vi "finding_high_and_low.vi"() -> ()   [LabVIEW 2019]
uses:
  Control.ctl
panel:
  in  "Stop":bool
  in  "Interrupt":bool
  out "Too low":bool
  out "Good":bool
  out "Too high":bool
  out "Value":dbl
  in  "Start":bool
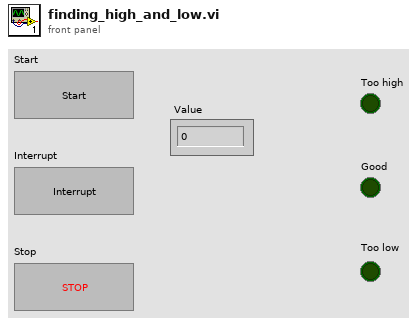
[diagram p1: front panel]
types:
  T1 = typedef "Control.ctl" = enum16{"measurment", "Good", "Too Low", "Too High", "End", "wait", "Pause"}
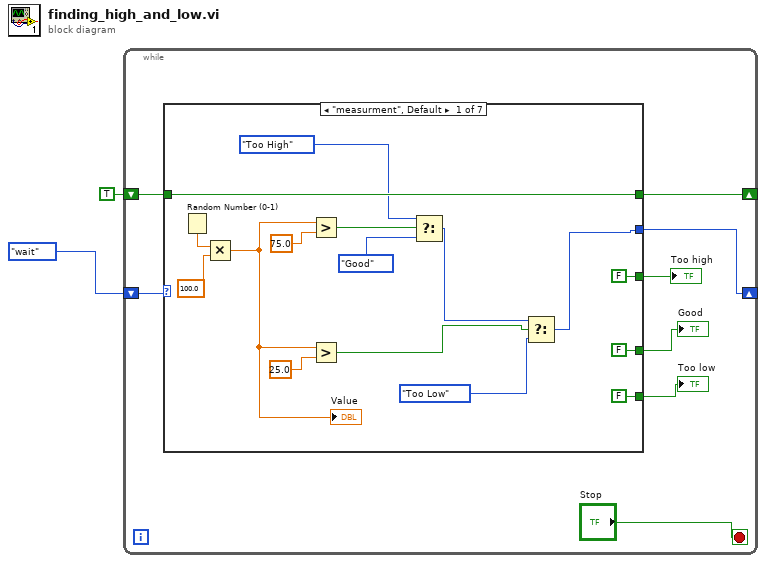
[diagram p0: block diagram]
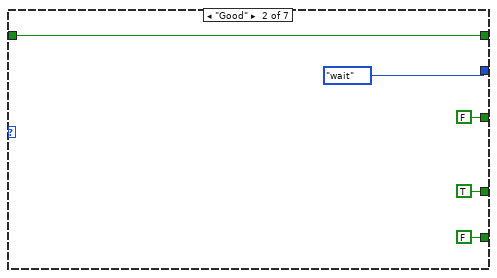
[diagram p2: hidden frame]
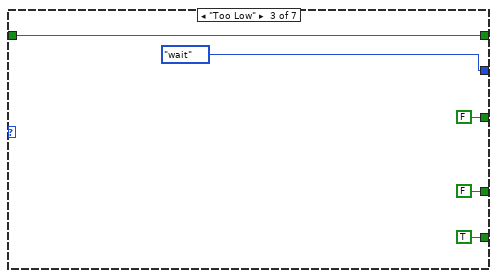
[diagram p3: hidden frame]
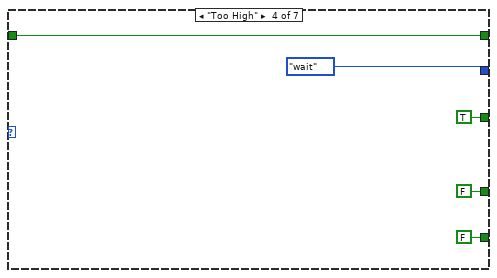
[diagram p4: hidden frame]
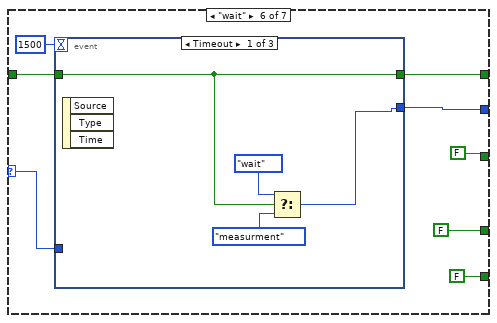
[diagram p6: hidden frame]
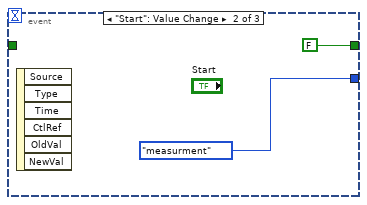
[diagram p7: hidden frame]
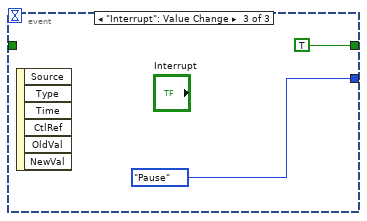
[diagram p8: hidden frame]
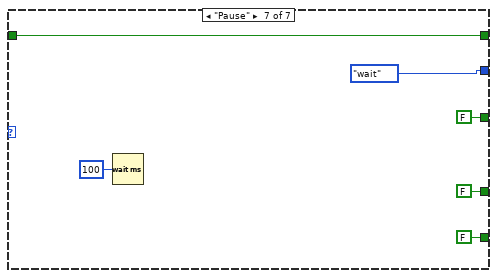
[diagram p9: hidden frame]
diagram:
  n1 = while {
    shift-right: [w9] -> _
    shift-left: Control."wait" -> [w10]
    shift-right: [w7] -> _
    shift-left: TRUE -> [w6]
    stop <- "Stop" stop-if-true
    n2 = case shown="\"measurment\", Default" w10 {
      selector: w10 -> [_ _ _ _ _ w44 _]
      tunnel: [w20 Control."wait" Control."wait" Control."wait" _ w50 Control."wait"] -> w9
      tunnel: [FALSE FALSE FALSE TRUE _ FALSE FALSE] -> w8
      tunnel: [w16 w31 w36 w41 w42 w48 w64] -> w7
      tunnel: w6 -> [w16 w31 w36 w41 w42 w47 w64]
      tunnel: [FALSE TRUE FALSE FALSE _ FALSE FALSE] -> w5
      tunnel: [FALSE FALSE TRUE FALSE _ FALSE FALSE] -> w4
      frame "measurment", Default {
        n3 = Random Number (0-1)() -> (number: 0 to 1=w12:dbl)
        n4 = Multiply(x=w12, y=100.0) -> (x*y=w13:dbl)
        "Value" <- w13
        n5 = Greater?(x=w13, y=75.0) -> (0:w23:bool)
        n6 = Greater?(x=w13, y=25.0) -> (0:w22:bool)
        n7 = Select(t=Control."Too High", s=w23, f=Control."Good") -> (s? t:f=w21:T1)
        n8 = Select(t=w21, s=w22, f=Control."Too Low") -> (s? t:f=w20:T1)
      }
      frame "Good" {
      }
      frame "Too Low" {
      }
      frame "Too High" {
      }
      frame "End" {
      }
      frame "wait" {
        n9 = event shown="[0] Timeout" {
          selector: _ -> [_ _ _]
          dyn-events: _ -> [_ _ _]
          timeout: 1500 -> [_ _ _]
          tunnel: [w51 Control."measurment" Control."Pause"] -> w50
          tunnel: [w54 FALSE TRUE] -> w48
          tunnel: w47 -> [w54 _ _]
          tunnel: w44 -> [_ _ _]
          event Timeout {
            n10 = event-data() -> ()  [unwired: 1 in, 3 out]
            n11 = Select(t=Control."wait", s=w54, f=Control."measurment") -> (s? t:f=w51:T1)
          }
          event "Start": Value Change {
            n12 = event-data() -> ()  [unwired: 1 in, 6 out]
          }
          event "Interrupt": Value Change {
            n13 = event-data() -> ()  [unwired: 1 in, 6 out]
          }
        }
      }
      frame "Pause" {
        n14 = Wait (ms)(milliseconds to wait=u32 100) -> ()  [unwired: 1 out]
      }
    }
    "Too high" <- w8
    "Good" <- w5
    "Too low" <- w4
  }
